vi "NegSignCheck.vi"(0 "regular expression":string, 1 "trimmed string":string) -> (2 "offset past match":i32, 3 "cc":string, 4 "bb":string, 5 "aa":string)   [LabVIEW 2014]
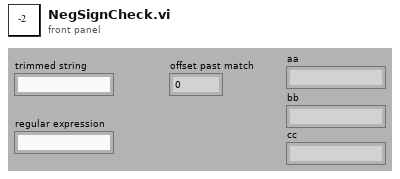
[diagram p1: front panel]
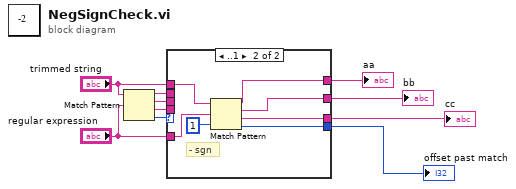
[diagram p0: block diagram]
diagram:
  n1 = Match Pattern(string="trimmed string", regular expression="regular expression") -> (before substring=w3:string, match substring=w2:string, after substring=w1:string, offset past match=w7:i32)  [unwired: 1 in]
  n2 = case shown="..1" w7 {
    selector: w7 -> [w14 _]
    tunnel: [w14 w18] -> w8
    tunnel: "trimmed string" -> [_ w21]
    tunnel: "regular expression" -> [_ w20]
    tunnel: [w13 w17] -> w6
    tunnel: [w12 w16] -> w5
    tunnel: [w11 w15] -> w4
    tunnel: w3 -> [w13 _]
    tunnel: w2 -> [w12 _]
    tunnel: w1 -> [w11 _]
    frame 2.. {
    }
    frame ..1 {
      # "- sgn"
      n3 = Match Pattern(string=w21, regular expression=w20, offset (0)=1) -> (before substring=w17:string, match substring=w16:string, after substring=w15:string, offset past match=w18:i32)
    }
  }
  "offset past match" <- w8
  "aa" <- w6
  "bb" <- w5
  "cc" <- w4
